vi "Split the String.vi"(5 "error in (no error)":errorcluster, 6 "Marker":string[](array[string])=["+", "-"], 7 "position":u32, 8 "string":string) -> (0 "error out":errorcluster, 1 "choice":string, 2 "new position":i32, 3 "after":string, 4 "before":string)   [LabVIEW 2020, in "NI_Gmath.lvlib"]
uses:
  <vilib>/gmath/NI_Gmath.lvlib
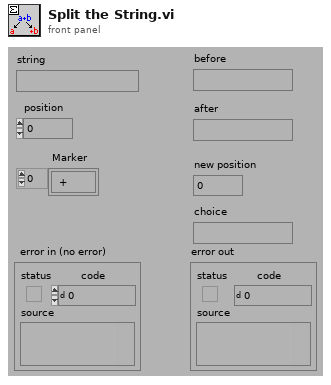
[diagram p1: front panel]
types:
  T1 = cluster{"status":bool, "offset of match":i32, "source":string}
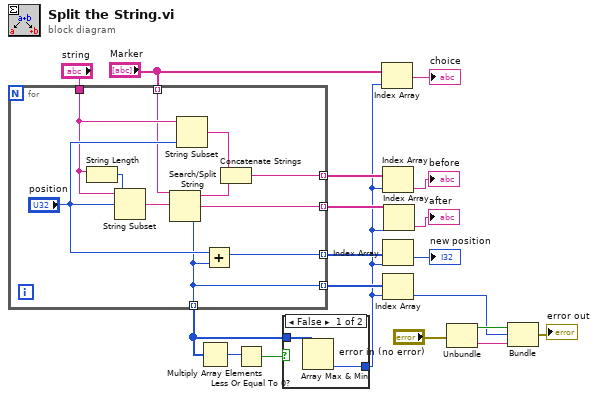
[diagram p0: block diagram]
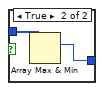
[diagram p2: hidden frame]
diagram:
  n1 = for {
    tunnel: "string" -> [w26]
    tunnel: "Marker" -> [w24] mode=indexing
    tunnel: [w20] -> w2 mode=indexing
    tunnel: [w23] -> w16 mode=indexing
    tunnel: [w22] -> w4 mode=indexing
    tunnel: [w21] -> w14 mode=indexing
    tunnel: [w20] -> w15 mode=indexing
    n2 = String Length(string=w26) -> (length=w29:i32)
    n3 = String Subset(string=w26, offset (0)="position", length (rest)=w29) -> (substring=w25:string)
    n4 = Search/Split String(string=w25, search string/char (-)=w24) -> (substring before match=w28:string, match + rest of string=w22:string, offset of match=w20:i32)  [unwired: 1 in]
    n5 = String Subset(string=w26, length (rest)="position") -> (substring=w27:string)  [unwired: 1 in]
    n6 = Add(x="position", y=w20) -> (x+y=w21:u32)
    n7 = Concatenate Strings(w27, w28) -> (w23:string)
  }
  n8 = Multiply Array Elements(1:w2) -> (0:w18:i32)
  n9 = Less Or Equal To 0?(x=w18) -> (x <= 0?=w17:bool)
  n10 = case shown="False" w17 {
    tunnel: w2 -> [w32 w34]
    tunnel: [w31 w33] -> w1
    frame False {
      n11 = Array Max & Min(array=w32) -> (min index (indices)=w31:i32)  [unwired: 3 out]
    }
    frame True {
      n12 = Array Max & Min(array=w34) -> (max index (indices)=w33:i32)  [unwired: 3 out]
    }
  }
  n13 = Index Array(array="Marker", index=w1) -> (element=→"choice":string)
  n14 = Index Array(array=w16, index=w1) -> (element=→"before":string)
  n15 = Index Array(array=w14, index=w1) -> (element=→"new position":u32)
  n16 = Index Array(array=w15, index=w1) -> (element=w5:i32)
  n17 = Index Array(array=w4, index=w1) -> (element=→"after":string)
  n18 = Unbundle("error in (no error)") -> ("status"=w8:bool, "source"=w7:string)  [unwired: 1 out]
  n19 = Bundle("status"=w8, "offset of match"=w5, "source"=w7) -> (→"error out":T1)  [unwired: 1 in]
